vi "Set Ref select window UI from file.vi"(8 "error in (no error)":errorcluster, 9 "Keys setup.DBL":T2, 10 "Section name":string, 11 "Refnum in":T1) -> (0 "error out":errorcluster, 3 "Refnum out":T1)   [LabVIEW 2017]
uses:
  Typedefs/Ini file interface (DBL).ctl
  <vilib>/Utility/config.llb/Config Data RefNum.ctl
  User Interface/Globals/gl_Windows Ctrl refs.vi
  <vilib>/Utility/config.llb/NI_LVConfig.lvlib
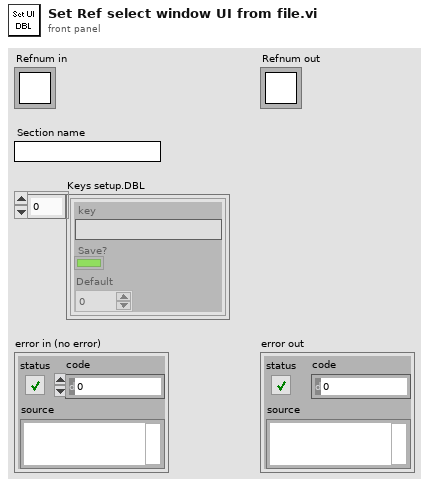
[diagram p1: front panel]
types:
  T1 = typedef "NI_LVConfig.lvlib/Config Data RefNum.ctl" = refnum<k1>
  T2 = typedef "Ini file interface (DBL).ctl" = cluster{"key":string, "Save?":bool, "Default":dbl}[]
  T3 = typedef "Ref select window ctrl refs.ctl" = cluster{"Channel Selector":refnum<vi>, "Boundary":refnum<vi>, "Image intensity":refnum<vi>}
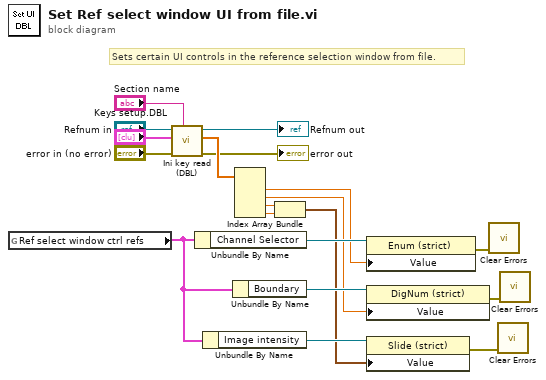
[diagram p0: block diagram]
diagram:
  # "Sets certain UI controls in the reference selection window from file."
  n1 = global read "gl_Windows Ctrl refs.vi" "Ref select window ctrl refs"() -> (w7:T3)
  n2 = call "Ini key read (DBL).vi"("Section name"="Section name", "error in (no error)"="error in (no error)", "Parameter names & setup"="Keys setup.DBL", "Ini file refnum in"="Refnum in") -> ("error out"=→"error out":errorcluster, "Value read/used"=w17:dbl[], "Ini file refnum out"=→"Refnum out":T1)  [unwired: 5 in]
  n3 = Unbundle By Name(w7) -> ("Channel Selector"=w12:refnum<vi>)
  n4 = Unbundle By Name(w7) -> ("Image intensity"=w10:refnum<vi>)
  n5 = Unbundle By Name(w7) -> ("Boundary"=w11:refnum<vi>)
  n6 = Index Array(array=w17) -> (element #1=w5:dbl, element #2=w4:dbl, element #3=w3:dbl, element #4=w2:dbl)  [unwired: 4 in]
  n7 = Bundle("value"=w3, "value"=w2) -> (w1:cluster{"value":dbl, "value":dbl})  [unwired: 1 in]
  n8 = property class="Enum (strict)"(reference=w12, "Value"=w5) -> (error out=w6:errorcluster)  [unwired: 1 in, 1 out]
  n9 = property class="DigNum (strict)"(reference=w11, "Value"=w4) -> (error out=w9:errorcluster)  [unwired: 1 in, 1 out]
  n10 = property class="Slide (strict)"(reference=w10, "Value"=w1) -> (error out=w8:errorcluster)  [unwired: 1 in, 1 out]
  n11 = call <vilib>:"Clear Errors.vi"("error in (no error)"=w6) -> ()  [unwired: 5 in, 2 out]
  n12 = call <vilib>:"Clear Errors.vi"("error in (no error)"=w8) -> ()  [unwired: 5 in, 2 out]
  n13 = call <vilib>:"Clear Errors.vi"("error in (no error)"=w9) -> ()  [unwired: 5 in, 2 out]
